vi "_openOrUseOpenStorage.vi"(4 "error in (no error)":errorcluster, 5 "function (open:0)":T1(ring), 7 "file path":path) -> (0 "error out":errorcluster, 3 "storage refnum":refnum<k20>)   [LabVIEW 2017]
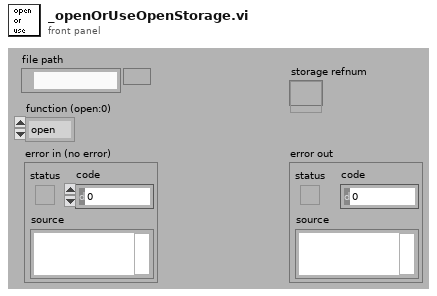
[diagram p1: front panel]
types:
  T1 = enum16{"open", "open or create", "create or replace", "create", "open (read only)"}
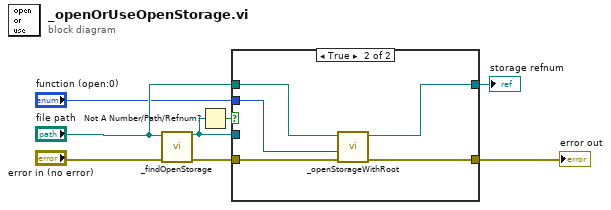
[diagram p0: block diagram]
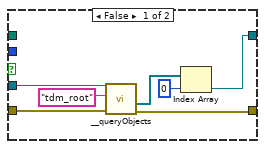
[diagram p2: hidden frame]
diagram:
  n1 = call <vilib>:"_findOpenStorage.vi"("error in (no error)"="error in (no error)", "Storage location"="file path") -> ("error out"=w6:errorcluster, "storage refnum"=w8:refnum<k20>)  [unwired: 4 in]
  n2 = Not A Number/Path/Refnum?(number/path/refnum=w8) -> (NaN/Path/Refnum?=w7:bool)
  n3 = case shown="True" w7 {
    tunnel: "function (open:0)" -> [_ w20]
    tunnel: [w11 w19] -> w2
    tunnel: [w10 w18] -> w3
    tunnel: "file path" -> [_ w17]
    tunnel: w6 -> [w12 w16]
    tunnel: w8 -> [w9 _]
    frame False {
      n4 = call <vilib>:"__queryObjects.vi"("error in (no error)"=w12, "Object type"="tdm_root" ("ObjectType"), "storage refnum"=w9) -> ("error out"=w11:errorcluster, "storage refnums"=w15:refnum<k20>[])  [unwired: 2 in, 1 out]
      n5 = Index Array(array=w15, index=0) -> (element=w10:refnum<k20>)
    }
    frame True {
      n6 = call <vilib>:"_openStorageWithRoot.vi"("error in (no error)"=w16, "Overwrite Options"=w20, "Storage Location"=w17) -> ("error out"=w19:errorcluster, "Data Object"=w18:refnum<k20>)  [unwired: 7 in]
    }
  }
  "storage refnum" <- w3
  "error out" <- w2
